vi "【抗扰】试验舱仿真器传递函数-带自然冷却.vi"() -> ()   [LabVIEW 2018]
panel:
  out "波形图表 2":dbl(graph)
  out "波形图表":cluster{"上限":dbl, "上限":dbl, "上限":dbl}(graph)
  in  "自然冷却按钮":bool
  out "1.8m试验仓仓内温度":dbl(graph)
  out "1.8m试验仓仓内压力":dbl(graph)=-0.0229152
  out "1M8仓温度仿真":dbl(slide)=73.625 scale=0.0..250.0
  out "1M8仓压力仿真":dbl(slide)=-0.0229152 scale=0.0..1.0
  out "压力":dbl
  out "f 5":dbl format="%.3f"
  out "d排气影响压力":dbl
  out "f 4":dbl format="%.3f"
  out "d进蒸汽影响压力":dbl
  out "f 3":dbl format="%.3f"
  out "d进空气影响压力":dbl
  out "f 2":dbl format="%.3f"
  out "d进空气影响温度":dbl
  out "f":dbl format="%.3f"
  out "d进蒸汽影响温度":dbl
  out "温度":dbl
  # "试验舱"
  # "压力"
  # "温度"
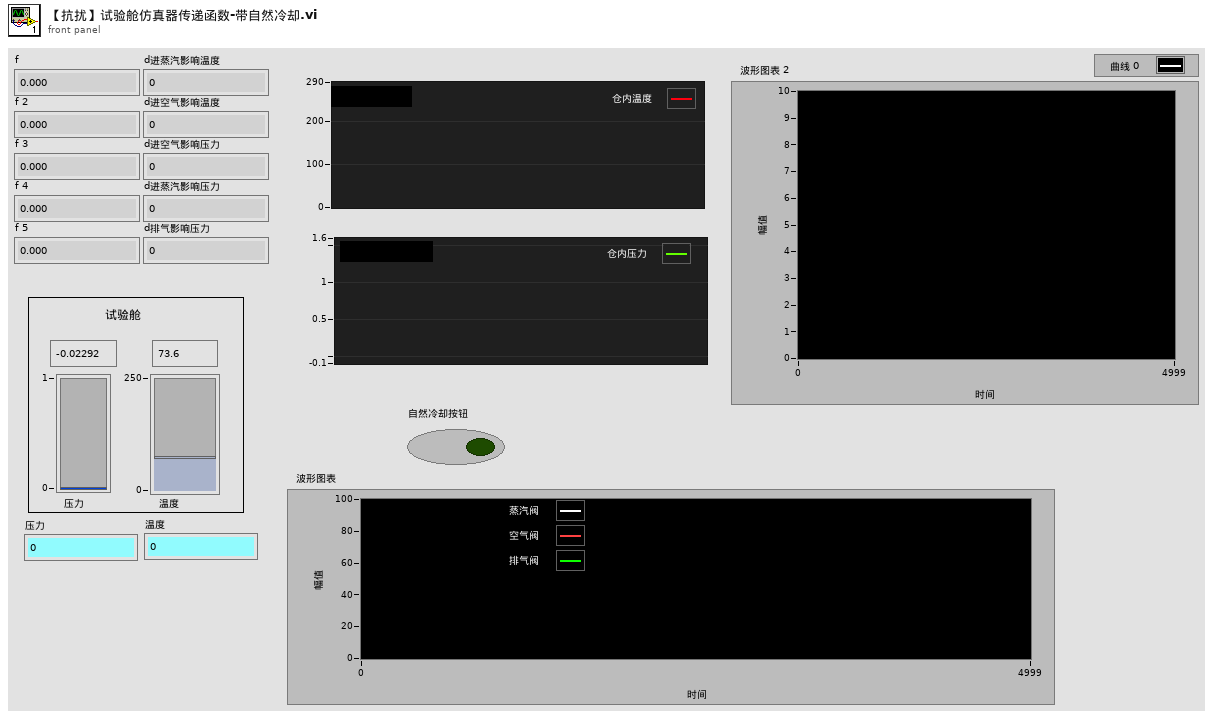
[diagram p1: front panel]
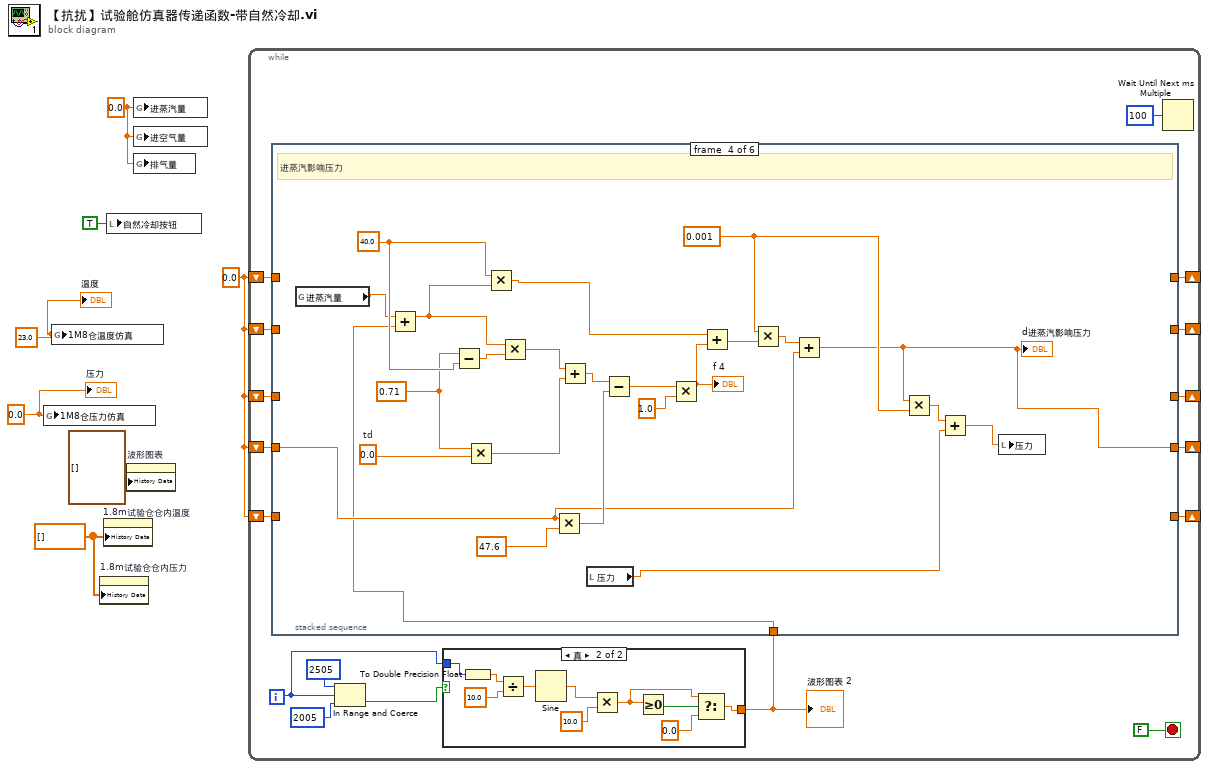
[diagram p0: block diagram]
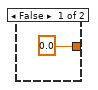
[diagram p2: hidden frame]
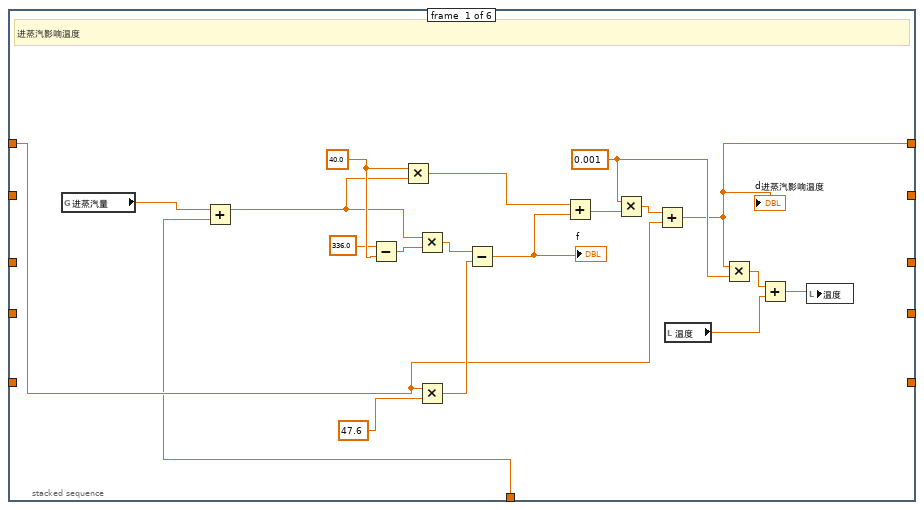
[diagram p3: hidden frame]
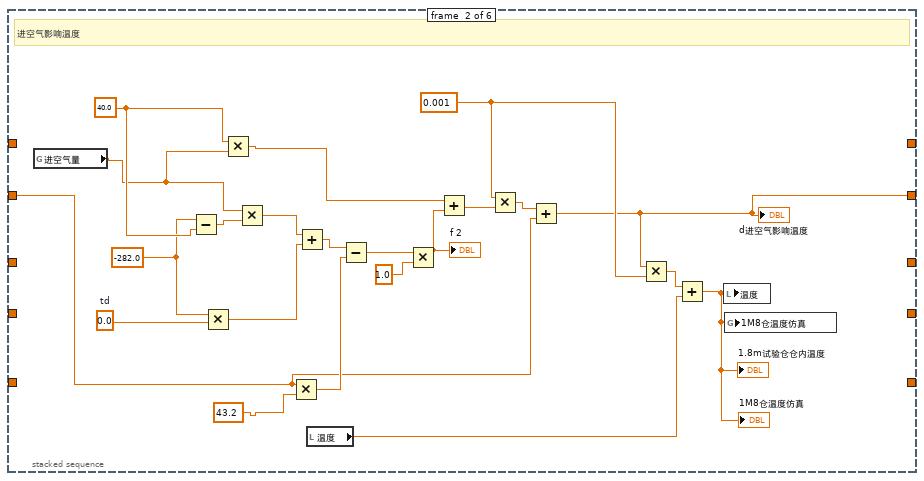
[diagram p4: hidden frame]
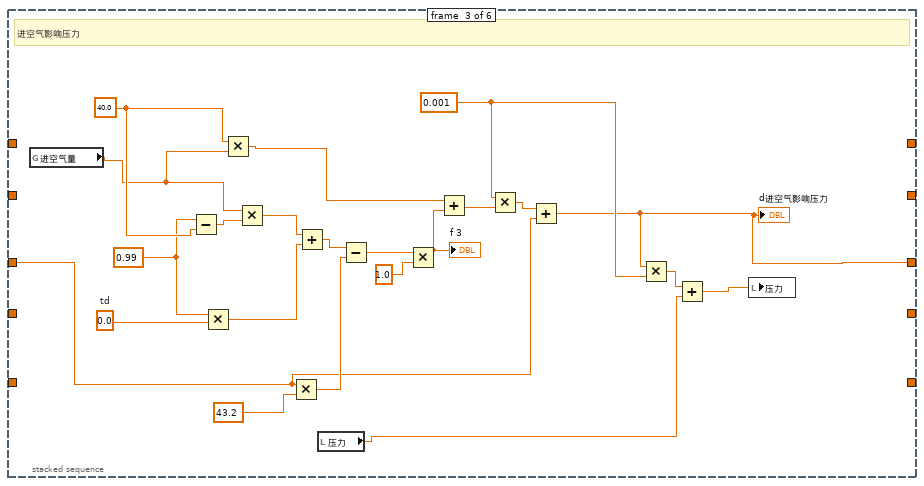
[diagram p5: hidden frame]
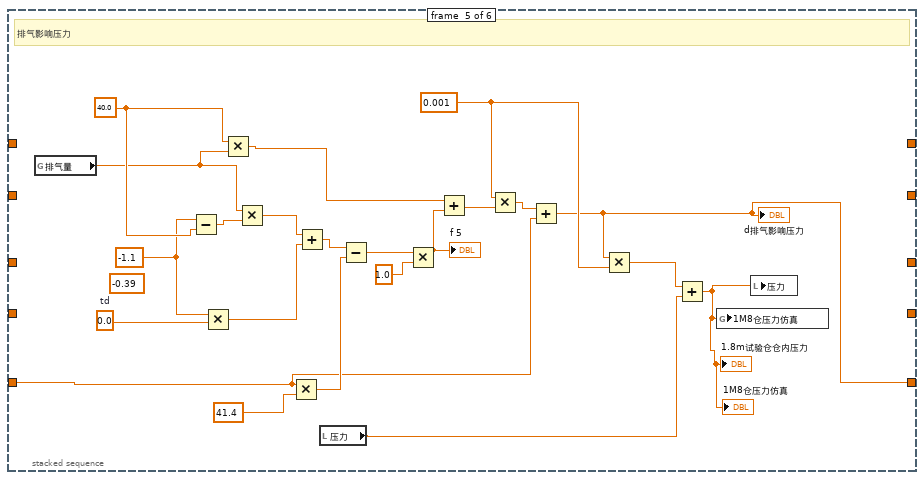
[diagram p6: hidden frame]
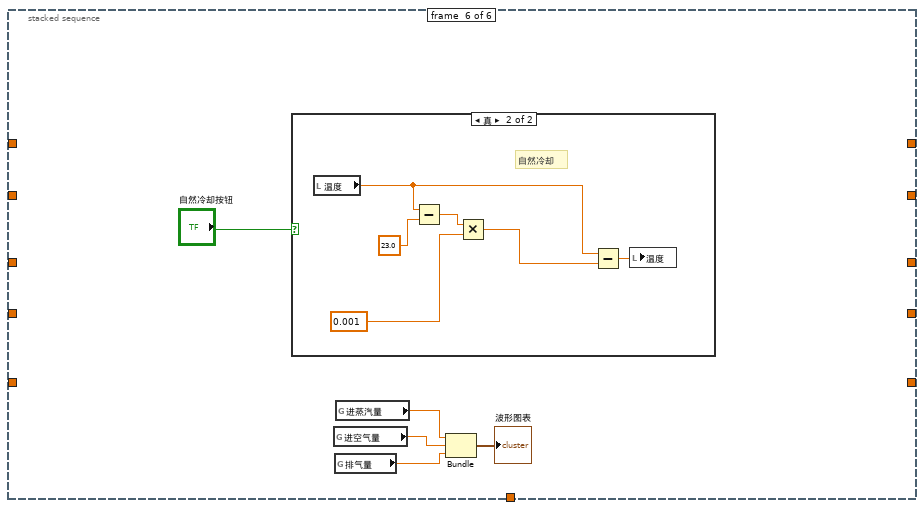
[diagram p7: hidden frame]
diagram:
  w3 = dbl[] [] ("历史数据")
  w6 = 0.0
  w7 = 0.0 ("进蒸汽量")
  w5 = 23.0 ("1.2m试验仓仓内温度")
  w4 = 0.0 ("1m2舱温度峰值")
  n1 = global write "全局变量.vi" "1M8仓压力仿真"(w4) -> ()
  n2 = global write "全局变量.vi" "1M8仓温度仿真"(w5) -> ()
  n3 = property on="1.8m试验仓仓内压力" class="WFChart (严格)"("History Data"=w3) -> ()  [unwired: 2 in, 2 out]
  n4 = property on="1.8m试验仓仓内温度" class="WFChart (严格)"("History Data"=w3) -> ()  [unwired: 2 in, 2 out]
  n5 = local write "自然冷却按钮"(TRUE ("自然冷却按钮")) -> ()
  n6 = property on="波形图表" class="WFChart (严格)"("History Data"=cluster{"上限":dbl, "上限":dbl, "上限":dbl}[] [] ("历史数据")) -> ()  [unwired: 2 in, 2 out]
  n7 = global write "全局变量.vi" "进蒸汽量"(w7) -> ()
  n8 = global write "全局变量.vi" "进空气量"(w7) -> ()
  n9 = global write "全局变量.vi" "排气量"(w7) -> ()
  n10 = while {
    shift-right: [w21] -> _
    shift-left: w6 -> [w22]
    shift-right: [w19] -> _
    shift-left: w6 -> [w20]
    shift-right: [w17] -> _
    shift-left: w6 -> [w18]
    shift-right: [w15] -> _
    shift-left: w6 -> [w16]
    shift-right: [w13] -> _
    shift-left: w6 -> [w14]
    i -> [w8]
    stop <- FALSE stop-if-true
    n11 = In Range and Coerce(upper limit=2505 ("上限"), x=w8, lower limit=2005 ("上限")) -> (In Range?=w10:bool)  [unwired: 1 out]
    n12 = case shown="真" w10 {
      tunnel: [0.0 w27] -> w9
      tunnel: w8 -> [_ w26]
      frame False {
      }
      frame True {
        n13 = To Double Precision Float(number=w26) -> (double precision float=w32:dbl)
        n14 = Divide(x=w32, y=10.0) -> (x/y=w31:dbl)
        n15 = Sine(x=w31) -> (sin(x)=w35:dbl)
        n16 = Multiply(x=w35, y=10.0) -> (x*y=w33:dbl)
        n17 = Greater Or Equal To 0?(x=w33) -> (x >= 0?=w34:bool)
        n18 = Select(t=w33, s=w34, f=0.0) -> (s? t:f=w27:dbl)
      }
    }
    "波形图表 2" <- w9
    n19 = stacked-sequence {
      tunnel: w22 -> [w42 _ _ _ _ _]
      tunnel: [w41 _ _ _ _ _] -> w21
      tunnel: w20 -> [_ w60 _ _ _ _]
      tunnel: [_ w59 _ _ _ _] -> w19
      tunnel: w18 -> [_ _ w83 _ _ _]
      tunnel: [_ _ w82 _ _ _] -> w17
      tunnel: w16 -> [_ _ _ w107 _ _]
      tunnel: [_ _ _ w106 _ _] -> w15
      tunnel: w14 -> [_ _ _ _ w129 _]
      tunnel: [_ _ _ _ w128 _] -> w13
      tunnel: w9 -> [w36 _ _ w99 _ _]
      frame #0 {
        w52 = 40.0 ("b0")
        w51 = 0.001
        # "进蒸汽影响温度"
        n20 = global read "全局变量.vi" "进蒸汽量"() -> (w53:dbl)
        n21 = Add(x=w53, y=w36) -> (x+y=w37:dbl)
        n22 = Subtract(x=336.0, y=w52) -> (x-y=w45:dbl)
        n23 = Multiply(x=w52, y=w37) -> (x*y=w44:dbl)
        n24 = Multiply(x=w37, y=w45) -> (x*y=w38:dbl)
        n25 = Multiply(x=w42, y=47.6) -> (x*y=w46:dbl)
        n26 = Subtract(x=w38, y=w46) -> (x-y=w50:dbl)
        "f" <- w50
        n27 = Add(x=w44, y=w50) -> (x+y=w49:dbl)
        n28 = Multiply(x=w51, y=w49) -> (x*y=w48:dbl)
        n29 = Add(x=w48, y=w42) -> (x+y=w41:dbl)
        "d进蒸汽影响温度" <- w41
        n30 = local read "温度"() -> (w54:dbl)
        n31 = Multiply(x=w41, y=w51) -> (x*y=w47:dbl)
        n32 = Add(x=w47, y=w54) -> (x+y=w43:dbl)
        n33 = local write "温度"(w43) -> ()
      }
      frame #1 {
        w75 = 0.0  # td
        w74 = 40.0 ("b0")
        w73 = 0.001
        w58 = -282.0 ("x")
        # "进空气影响温度"
        n34 = global read "全局变量.vi" "进空气量"() -> (w56:dbl)
        n35 = Subtract(x=w58, y=w74) -> (x-y=w62:dbl)
        n36 = Multiply(x=w58, y=w75) -> (x*y=w64:dbl)
        n37 = Multiply(x=w74, y=w56) -> (x*y=w61:dbl)
        n38 = Multiply(x=w56, y=w62) -> (x*y=w63:dbl)
        n39 = Multiply(x=w60, y=43.2) -> (x*y=w66:dbl)
        n40 = Add(x=w63, y=w64) -> (x+y=w65:dbl)
        n41 = local read "温度"() -> (w76:dbl)
        n42 = Subtract(x=w65, y=w66) -> (x-y=w67:dbl)
        n43 = Multiply(x=w67, y=1.0) -> (x*y=w71:dbl)
        "f 2" <- w71
        n44 = Add(x=w61, y=w71) -> (x+y=w70:dbl)
        n45 = Multiply(x=w73, y=w70) -> (x*y=w69:dbl)
        n46 = Add(x=w69, y=w60) -> (x+y=w59:dbl)
        "d进空气影响温度" <- w59
        n47 = Multiply(x=w59, y=w73) -> (x*y=w68:dbl)
        n48 = Add(x=w68, y=w76) -> (x+y=w55:dbl)
        "1.8m试验仓仓内温度" <- w55
        "1M8仓温度仿真" <- w55
        n49 = local write "温度"(w55) -> ()
        n50 = global write "全局变量.vi" "1M8仓温度仿真"(w55) -> ()
      }
      frame #2 {
        w98 = 0.0  # td
        w97 = 40.0 ("b0")
        w96 = 0.001
        w81 = 0.99 ("x")
        # "进空气影响压力"
        n51 = global read "全局变量.vi" "进空气量"() -> (w79:dbl)
        n52 = Subtract(x=w81, y=w97) -> (x-y=w85:dbl)
        n53 = Multiply(x=w81, y=w98) -> (x*y=w87:dbl)
        n54 = Multiply(x=w97, y=w79) -> (x*y=w84:dbl)
        n55 = Multiply(x=w79, y=w85) -> (x*y=w86:dbl)
        n56 = Multiply(x=w83, y=43.2) -> (x*y=w89:dbl)
        n57 = Add(x=w86, y=w87) -> (x+y=w88:dbl)
        n58 = local read "压力"() -> (w78:dbl)
        n59 = Subtract(x=w88, y=w89) -> (x-y=w90:dbl)
        n60 = Multiply(x=w90, y=1.0) -> (x*y=w94:dbl)
        "f 3" <- w94
        n61 = Add(x=w84, y=w94) -> (x+y=w93:dbl)
        n62 = Multiply(x=w96, y=w93) -> (x*y=w92:dbl)
        n63 = Add(x=w92, y=w83) -> (x+y=w82:dbl)
        "d进空气影响压力" <- w82
        n64 = Multiply(x=w82, y=w96) -> (x*y=w91:dbl)
        n65 = Add(x=w91, y=w78) -> (x+y=w77:dbl)
        n66 = local write "压力"(w77) -> ()
      }
      frame #3 {
        w122 = 0.0  # td
        w121 = 40.0 ("b0")
        w120 = 0.001
        w105 = 0.71 ("x")
        # "进蒸汽影响压力"
        n67 = global read "全局变量.vi" "进蒸汽量"() -> (w103:dbl)
        n68 = Add(x=w103, y=w99) -> (x+y=w100:dbl)
        n69 = Subtract(x=w105, y=w121) -> (x-y=w109:dbl)
        n70 = Multiply(x=w105, y=w122) -> (x*y=w111:dbl)
        n71 = Multiply(x=w121, y=w100) -> (x*y=w108:dbl)
        n72 = Multiply(x=w100, y=w109) -> (x*y=w110:dbl)
        n73 = Multiply(x=w107, y=47.6) -> (x*y=w113:dbl)
        n74 = Add(x=w110, y=w111) -> (x+y=w112:dbl)
        n75 = local read "压力"() -> (w102:dbl)
        n76 = Subtract(x=w112, y=w113) -> (x-y=w114:dbl)
        n77 = Multiply(x=w114, y=1.0) -> (x*y=w118:dbl)
        "f 4" <- w118
        n78 = Add(x=w108, y=w118) -> (x+y=w117:dbl)
        n79 = Multiply(x=w120, y=w117) -> (x*y=w116:dbl)
        n80 = Add(x=w116, y=w107) -> (x+y=w106:dbl)
        "d进蒸汽影响压力" <- w106
        n81 = Multiply(x=w106, y=w120) -> (x*y=w115:dbl)
        n82 = Add(x=w115, y=w102) -> (x+y=w101:dbl)
        n83 = local write "压力"(w101) -> ()
      }
      frame #4 {
        (unwired) -0.39 ("x")
        w144 = 0.0  # td
        w143 = 40.0 ("b0")
        w142 = 0.001
        w127 = -1.1 ("x")
        # "排气影响压力"
        n84 = global read "全局变量.vi" "排气量"() -> (w125:dbl)
        n85 = Subtract(x=w127, y=w143) -> (x-y=w131:dbl)
        n86 = Multiply(x=w127, y=w144) -> (x*y=w133:dbl)
        n87 = Multiply(x=w143, y=w125) -> (x*y=w130:dbl)
        n88 = Multiply(x=w125, y=w131) -> (x*y=w132:dbl)
        n89 = Multiply(x=w129, y=41.4) -> (x*y=w135:dbl)
        n90 = Add(x=w132, y=w133) -> (x+y=w134:dbl)
        n91 = local read "压力"() -> (w124:dbl)
        n92 = Subtract(x=w134, y=w135) -> (x-y=w136:dbl)
        n93 = Multiply(x=w136, y=1.0) -> (x*y=w140:dbl)
        "f 5" <- w140
        n94 = Add(x=w130, y=w140) -> (x+y=w139:dbl)
        n95 = Multiply(x=w142, y=w139) -> (x*y=w138:dbl)
        n96 = Add(x=w138, y=w129) -> (x+y=w128:dbl)
        "d排气影响压力" <- w128
        n97 = Multiply(x=w128, y=w142) -> (x*y=w137:dbl)
        n98 = Add(x=w137, y=w124) -> (x+y=w123:dbl)
        "1M8仓压力仿真" <- w123
        "1.8m试验仓仓内压力" <- w123
        n99 = global write "全局变量.vi" "1M8仓压力仿真"(w123) -> ()
        n100 = local write "压力"(w123) -> ()
      }
      frame #5 {
        n101 = case shown="真" "自然冷却按钮" {
          frame False {
          }
          frame True {
            # "自然冷却"
            n102 = local read "温度"() -> (w154:dbl)
            n103 = Subtract(x=w154, y=23.0) -> (x-y=w152:dbl)
            n104 = Multiply(x=w152, y=0.001) -> (x*y=w150:dbl)
            n105 = Subtract(x=w154, y=w150) -> (x-y=w155:dbl)
            n106 = local write "温度"(w155) -> ()
          }
        }
        n107 = global read "全局变量.vi" "进空气量"() -> (w146:dbl)
        n108 = global read "全局变量.vi" "排气量"() -> (w145:dbl)
        n109 = global read "全局变量.vi" "进蒸汽量"() -> (w147:dbl)
        n110 = Bundle("进蒸汽量"=w147, "进空气量"=w146, "排气量"=w145) -> (→"波形图表":cluster{"进蒸汽量":dbl, "进空气量":dbl, "排气量":dbl})  [unwired: 1 in]
      }
    }
    n111 = Wait Until Next ms Multiple(millisecond multiple=u32 100) -> ()  [unwired: 1 out]
  }
  "温度" <- w5
  "压力" <- w4
